vi "Planar Three Body Problem.vi"() -> ()   [LabVIEW 2023]
doc: "Demonstrates the use of the ODE Cash Karp 5th Order VI to solve the equations of motion for the Planar-Three-Body problem."
uses:
  <vilib>/Analysis/1siggen.llb/Ramp Pattern by Delta.vi
  <vilib>/gmath/NI_Gmath.lvlib
  <vilib>/Analysis/NI_AALBase.lvlib
panel:
  out "time":dbl
  in  "Table":string[][](table)=[["p0", "r0", "1"], ["q0", "s0", "-1"], ["r0", "M1*(p1-p0)/sqrt((p1-p0)^2+(q1-q0)^2)^3+M2*(p2-p0)/sqrt((p2-p0)^2+(q2-q0)^2)^3", "0"], ["s0", "M1*(q1-q0)/sqrt((p1-p0)^2+(q1-q0)^2)^3+M2*(q2-q0)/sqrt((p2-p0)^2+(q2-q0)^2)^3", "0"], ["p1", "r1", "1"], ["q1", "s1", "3"], ["r1", "M2*(p2-p1)/sqrt((p2-p1)^2+(q2-q1)^2)^3+M0*(p0-p1)/sqrt((p0-p1)^2+(q0-q1)^2)^3", "0"], ["s1", "M2*(q2-q1)/sqrt((p2-p1)^2+(q2-q1)^2)^3+M0*(q0-q1)/sqrt((p0-p1)^2+(q0-q1)^2)^3", "0"], ["p2", "r2", "-2"], ["q2", "s2", "-1"], ["r2", "M0*(p0-p2)/sqrt((p0-p2)^2+(q0-q2)^2)^3+M1*(p1-p2)/sqrt((p1-p2)^2+(q1-q2)^2)^3", "0"], ["s2", "M0*(q0-q2)/sqrt((p0-p2)^2+(q0-q2)^2)^3+M1*(q1-q2)/sqrt((p1-p2)^2+(q1-q2)^2)^3", "0"]]
  in  "m0":dbl=5.0 min=0.01
  in  "m1":dbl=3.0 min=0.01
  in  "m2":dbl=4.0 min=0.01
  in  "time end":dbl=10.0 min=0.0
  in  "h":dbl=0.001 min=1e-20 format="%0.1e"
  out "movement of three bodies":T1(graph)
  # "Overview: Demonstrates the use of ODE Cash Karp 5th Order VI to solve the equations of motion for the Planar-Three-Body problem.\nRequirements: LabVIEW Full Development System\nInstructions:\nRun the VI."
  # "See the block diagram for the theory behind these formulas."
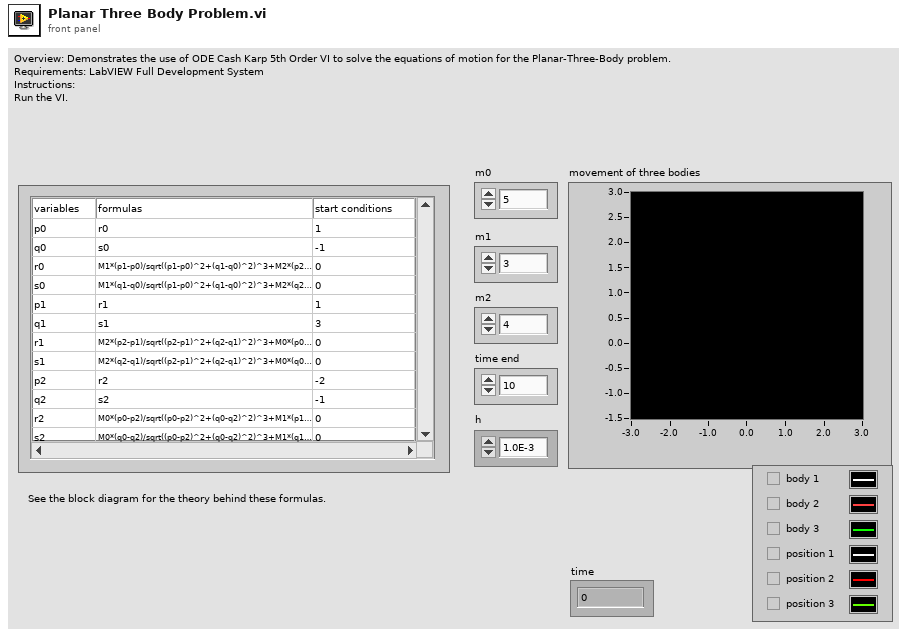
[diagram p1: front panel]
types:
  T1 = cluster{"X Values (solution)":dbl[], "X Values (solution)":dbl[]}[]
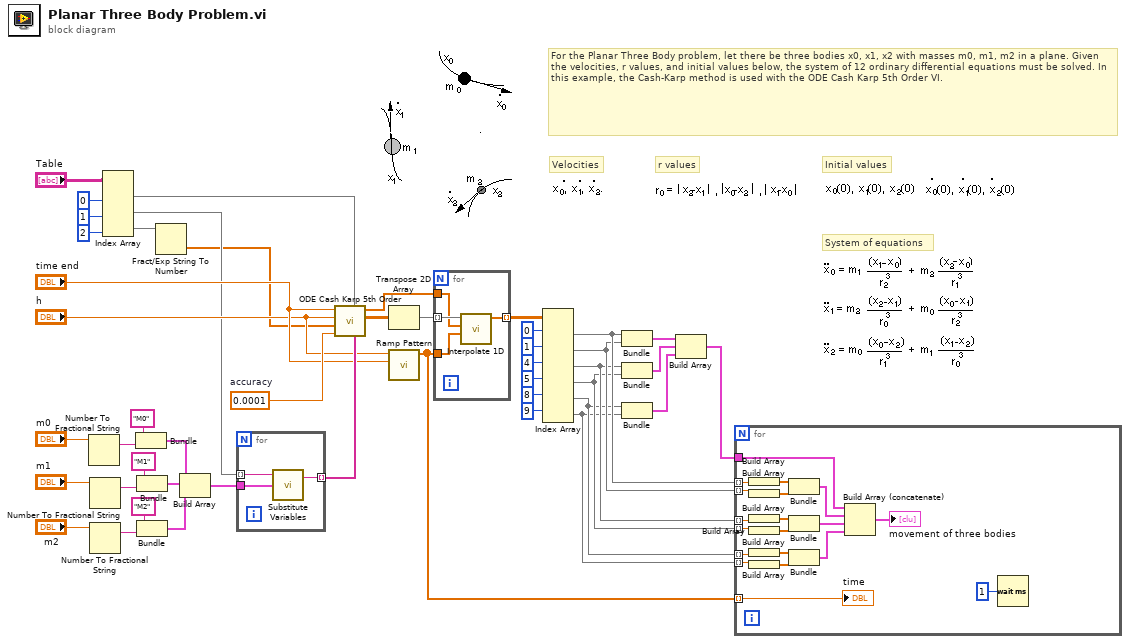
[diagram p0: block diagram]
diagram:
  w42 = 0.0001  # accuracy
  # "System of equations"
  # "Initial values"
  # "r values"
  # "Velocities"
  # "For the Planar Three Body problem, let there be three bodies x0, x1, x2 with masses m0, m1, m2 in a plane. Given the velocities, r values, and initial values below, the system of 12 ordinary differential equations must be solved. In this example, the Cash-Karp method is used with the ODE Cash Karp 5th Order VI."
  n1 = Number To Fractional String(number="m0") -> (F-format string=w41:string)  [unwired: 3 out]
  n2 = Number To Fractional String(number="m1") -> (F-format string=w38:string)  [unwired: 3 out]
  n3 = Number To Fractional String(number="m2") -> (F-format string=w37:string)  [unwired: 3 out]
  n4 = Index Array(array="Table", index (col) #1=0 ("disabled index (col)"), index (col) #2=1 ("index (col)"), index (col) #3=2 ("index (col)")) -> (element #1=w6:string[], element #2=w7:string[], element #3=w3:string[])  [unwired: 3 in]
  n5 = Bundle("M0", w41) -> (w35:cluster{string, string})  [unwired: 1 out]
  n6 = Bundle("M1", w38) -> (w34:cluster{string, string})  [unwired: 1 out]
  n7 = Bundle("M2", w37) -> (w33:cluster{string, string})  [unwired: 1 out]
  n8 = Fract/Exp String To Number(string=w3) -> (number=w2:dbl[])  [unwired: 3 in, 1 out]
  n9 = Build Array(w35, w34, w33) -> (w32:cluster{string, string}[])
  n10 = for {
    tunnel: w7 -> [w49] mode=indexing
    tunnel: w32 -> [w47]
    tunnel: [w48] -> w46 mode=indexing
    n11 = call <vilib>:"Substitute Variables.vi"("Substitution Rules"=w47, "original formula"=w49) -> ("formula after substitution"=w48:string)  [unwired: 1 in, 1 out]
  }
  n12 = call <vilib>:"ODE Cash Karp 5th Order.vi"("F(X,t) (right sides of the ODE\nas functions of X and t)"=w46, "X (name of variables)"=w6, "accuracy"=w42, "X0"=w2, "h (step rate)"="h", "time end"="time end") -> ("X Values (solution)"=w21:dbl[][], "Times"=w13:dbl[])  [unwired: 2 in, 2 out]
  n13 = Transpose 2D Array(2D array=w21) -> (transposed array=w12:dbl[][])
  n14 = call-poly <vilib>:"Ramp Pattern.vi"("end"="time end", "delta"="h") -> ("Ramp Pattern"=w1:dbl[])  [unwired: 7 in, 2 out]
  n15 = for {
    tunnel: w12 -> [w53] mode=indexing
    tunnel: [w52] -> w20 mode=indexing
    tunnel: w13 -> [w51]
    tunnel: w1 -> [w50]
    n16 = call <vilib>:"Interpolate 1D.vi"("xi"=w50, "X"=w51, "Y"=w53) -> ("yi"=w52:dbl[])  [unwired: 6 in, 2 out]
  }
  n17 = Index Array(array=w20, index (row) #1=0 ("disabled index (col)"), index (row) #2=1 ("index (col)"), index (row) #3=4 ("index (col)"), index (row) #4=5 ("index (col)"), index (row) #5=8 ("index (col)"), index (row) #6=9 ("index (col)")) -> (element #1=w28:dbl[], element #2=w27:dbl[], element #3=w26:dbl[], element #4=w25:dbl[], element #5=w24:dbl[], element #6=w23:dbl[])  [unwired: 6 in]
  n18 = Bundle("yi"=w28, "yi"=w27) -> (w45:cluster{"yi":dbl[], "yi":dbl[]})  [unwired: 1 out]
  n19 = Bundle("yi"=w26, "yi"=w25) -> (w44:cluster{"yi":dbl[], "yi":dbl[]})  [unwired: 1 out]
  n20 = Bundle("yi"=w24, "yi"=w23) -> (w43:cluster{"yi":dbl[], "yi":dbl[]})  [unwired: 1 out]
  n21 = Build Array(w45, w44, w43) -> (w22:cluster{"yi":dbl[], "yi":dbl[]}[])
  n22 = for {
    tunnel: w28 -> [w72] mode=indexing
    tunnel: w27 -> [w71] mode=indexing
    tunnel: w26 -> [w64] mode=indexing
    tunnel: w25 -> [w63] mode=indexing
    tunnel: w24 -> [w62] mode=indexing
    tunnel: w23 -> [w61] mode=indexing
    tunnel: w22 -> [w57]
    tunnel: w1 -> [w54] mode=indexing
    n23 = Build Array(w72) -> (w70:dbl[])
    n24 = Build Array(w71) -> (w69:dbl[])
    n25 = Build Array(w64) -> (w67:dbl[])
    n26 = Build Array(w63) -> (w68:dbl[])
    n27 = Build Array(w62) -> (w66:dbl[])
    n28 = Build Array(w61) -> (w65:dbl[])
    n29 = Bundle(w70, w69) -> (w60:cluster{dbl[], dbl[]})  [unwired: 1 out]
    n30 = Bundle(w67, w68) -> (w59:cluster{dbl[], dbl[]})  [unwired: 1 out]
    n31 = Bundle(w66, w65) -> (w58:cluster{dbl[], dbl[]})  [unwired: 1 out]
    n32 = Build Array (concatenate)(w57, w60, w59, w58) -> (→"movement of three bodies":cluster{"yi":dbl[], "yi":dbl[]}[])
    n33 = Wait (ms)(milliseconds to wait=u32 1) -> ()  [unwired: 1 out]
    "time" <- w54
  }
